vi "Latitud.vi"() -> ()   [LabVIEW 2014]
panel:
  out "Numeric":dbl
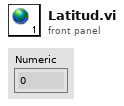
[diagram p1: front panel]
diagram:
